vi "CorrectDistance.vi"(3 "CenterPoint":dbl=24.0 format="%#_13g", 5 "Distance":dbl=29.337500000000006 format="%#_13g") -> (19 "In Range?":bool, 21 "Right Motor":dbl=0.4 format="%#_13g", 22 "Left Motor":dbl=0.4 format="%#_13g")   [LabVIEW 2016]
panel:
  in  "Speed":dbl=0.5 format="%#_13g"
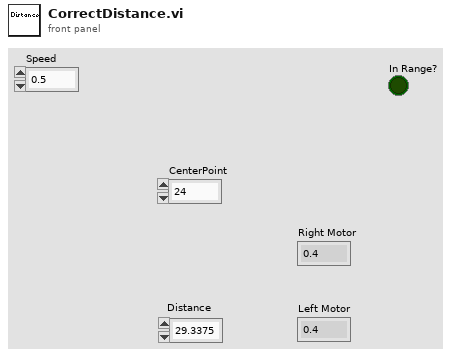
[diagram p1: front panel]
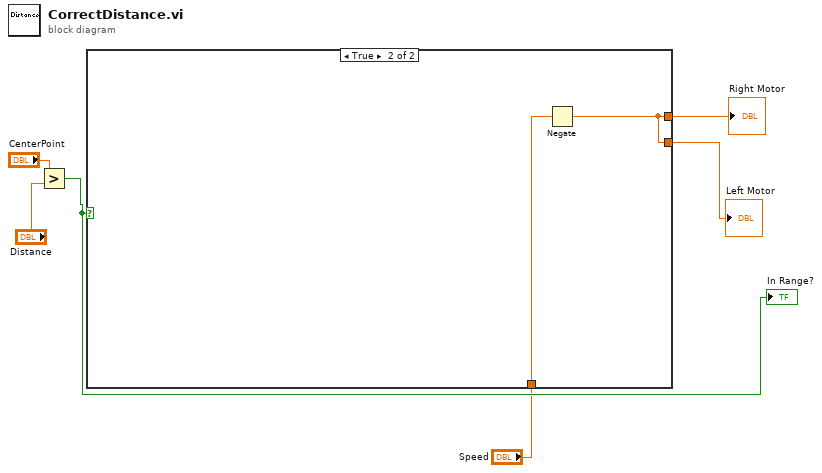
[diagram p0: block diagram]
diagram:
  n1 = Greater?(x="CenterPoint", y="Distance") -> (0:w2:bool)
  "In Range?" <- w2
  n2 = case shown="True" w2 {
    tunnel: [w7 w8] -> w4
    tunnel: [w7 w8] -> w3
    tunnel: "Speed" -> [w7 w9]
    frame False {
    }
    frame True {
      n3 = Negate(x=w9) -> (-x=w8:dbl)
    }
  }
  "Right Motor" <- w4
  "Left Motor" <- w3
